vi "Init Core.vi"(8 "error in (no error)":errorcluster, 11 "uPlugin_Handler in":refnum<class "uPlugin_Handler.lvclass">) -> (0 "error out":errorcluster, 3 "uPlugin_Handler":refnum<class "uPlugin_Handler.lvclass">)   [LabVIEW 2021, in "uPlug.lvlib" / "uPlugin_Handler.lvclass"]
doc: "Dynamic dispatch method to initialize the plugin handler."
uses:
  uPlugin_Handler.lvclass
  uPlugin_Handler.lvclass/uPlugin_Handler.ctl
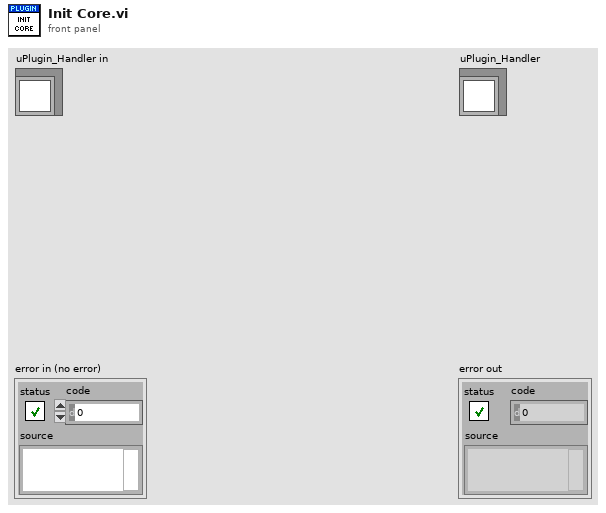
[diagram p1: front panel]
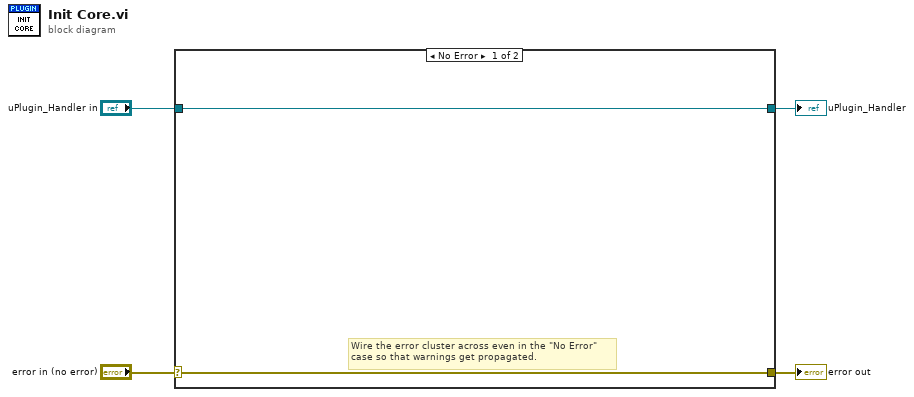
[diagram p0: block diagram]
diagram:
  n1 = case shown="No Error" "error in (no error)" {
    selector: "error in (no error)" -> [w5 w8]
    tunnel: [w5 w8] -> w3
    tunnel: [w6 w7] -> w1
    tunnel: "uPlugin_Handler in" -> [w6 w7]
    frame No Error {
      # "Wire the error cluster across even in the \"No Error\"\ncase so that warnings get propagated."
    }
    frame Error {
    }
  }
  "error out" <- w3
  "uPlugin_Handler" <- w1
